vi "Tegam4040 -- SetInputImpedance.vi"(8 "error in (no error)":errorcluster, 10 "Input Impedance":enum16{" 1 MOhm", "50 Ohm"}(ring), 11 "Instrument Session Handle In":u32 format="%x") -> (0 "error out":errorcluster, 3 "Instrument Session Handle Out (dupl)":u32 format="%x")   [LabVIEW 2010]
panel:
  out "VISA Error Code":i32 format="%x"
  out "Tegam Error Code":i32
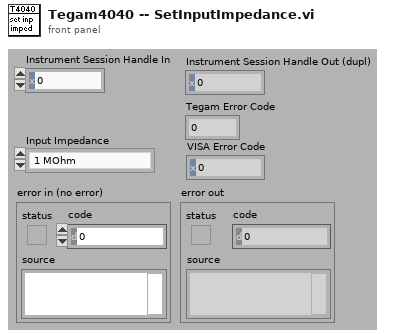
[diagram p1: front panel]
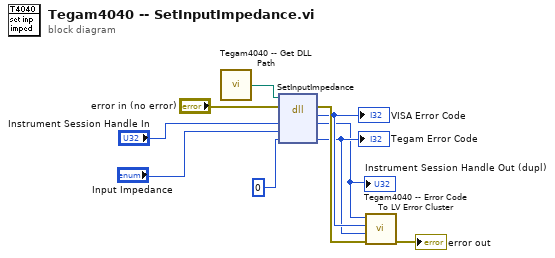
[diagram p0: block diagram]
diagram:
  n1 = call "Tegam4040 -- Get DLL Path.vi"() -> ("DLL Path"=w7:path)  [unwired: 8 in]
  n2 = dll-call lib="C:/Documents and Settings/Administrator/My Documents/Visual Studio 2005/Projects/Tegam4040CDriver/debug/Tegam4040CDriver.dll" fn="SetInputImpedance" ("Tegam4040CDriver.dll:Close4040")(path in=w7, error in="error in (no error)", "instrSession"="Instrument Session Handle In", "inputImpedance"="Input Impedance", "tegamError"=0) -> (error out=w9:errorcluster, "status"=w5:i32, "instrSession"=w2:u32, "tegamError"=w4:i32)  [unwired: 2 in, 1 out]
  "Tegam Error Code" <- w4
  "VISA Error Code" <- w5
  "Instrument Session Handle Out (dupl)" <- w2
  n3 = call "Tegam4040 -- Error Code To LV Error Cluster.vi"("error in (no error)"=w9, "Driver Error Code"=w4, "VISA Error Code"=w5, "Instrument Session Handle"=w2) -> ("error out"=→"error out":errorcluster)  [unwired: 7 in]
